vi "direct_tcpip.vi"() -> ()   [LabVIEW 2013]
uses:
  <vilib>/Utility/error.llb/DialogType.ctl
  libssh2/libssh2_init_default.vi
  libssh2/libssh2_session_handshake_tcp.vi
  libssh2/libssh2.lvlib
panel:
  in  "stop":bool
  out "error out":errorcluster
  in  "remote_destport":i32=2222
  in  "remote_desthost":string="localhost"
  in  "local_listenport":u16=4444
  in  "local_listenip":string="localhost"
  in  "server_ip":string="127.0.0.1"
  in  "password":string
  in  "username":string
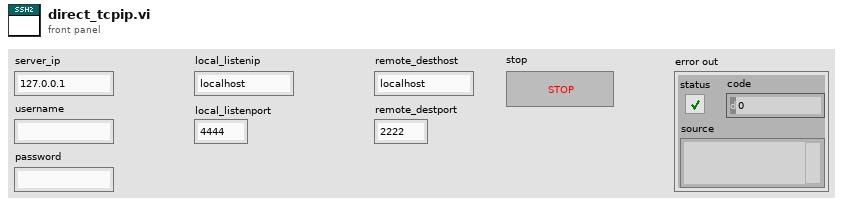
[diagram p1: front panel]
types:
  T1 = typedef "libssh2.lvlib/Session Refnum.ctl" = refnum<k1>
  T2 = typedef "libssh2.lvlib/Channel Refnum.ctl" = refnum<k1>
  T3 = enum16{"Standard", "Buffered", "CRLF", "Immediate"}
  T4 = typedef "DialogType.ctl" = u16
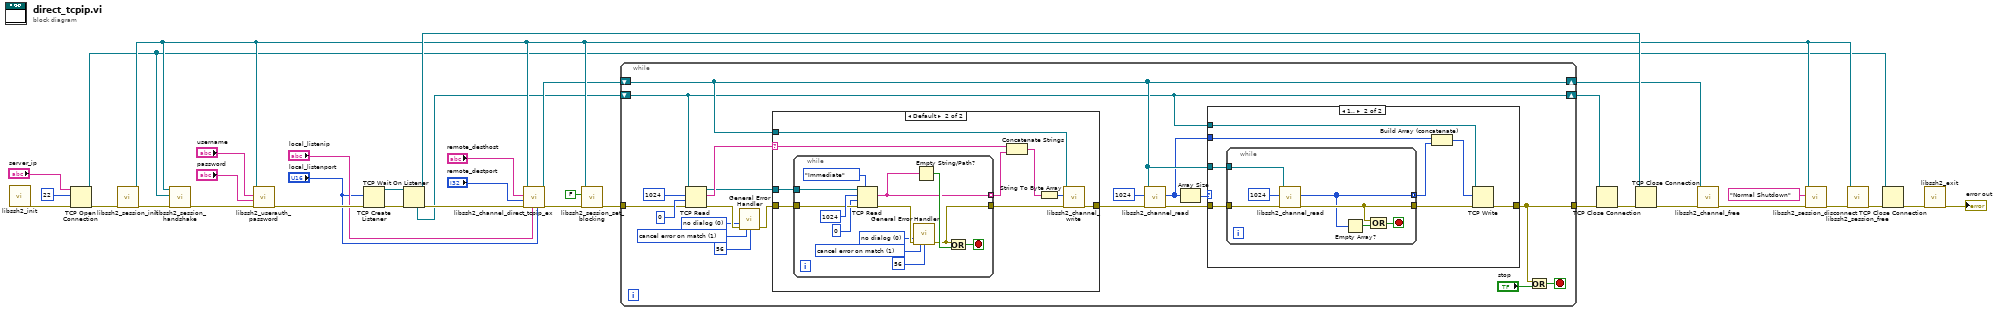
[diagram p0: block diagram]
diagram:
  n1 = call-poly "libssh2_init.vi"() -> ("error out"=w35:errorcluster)  [unwired: 11 in]
  n2 = TCP Open Connection(address="server_ip", remote port or service name=u16 22, error in (no error)=w35) -> (connection ID=w2:refnum<k5>, error out=w32:errorcluster)  [unwired: 2 in]
  n3 = call "libssh2_session_init.vi"("error in (no error)"=w32) -> ("error out"=w1:errorcluster, "session"=w18:T1)  [unwired: 9 in]
  n4 = call-poly "libssh2_session_handshake.vi"("error in (no error)"=w1, "tcp connection"=w2, "session"=w18) -> ("error out"=w31:errorcluster)  [unwired: 8 in]
  n5 = call "libssh2_userauth_password.vi"("error in (no error)"=w31, "password"="password", "username"="username", "session"=w18) -> ("error out"=w30:errorcluster)  [unwired: 7 in]
  n6 = TCP Create Listener(8:w30, 10:"local_listenport") -> (0:w17:errorcluster, 3:w12:refnum<k5>)  [unwired: 3 in, 1 out]
  n7 = TCP Wait On Listener(8:w17, 11:w12) -> (0:w27:errorcluster, 3:w19:refnum<k5>, 4:w5:refnum<k5>)  [unwired: 2 in, 2 out]
  n8 = call "libssh2_channel_direct_tcpip_ex.vi"("sport"="local_listenport", "shost"="local_listenip", "error in (no error)"=w27, "port"="remote_destport", "host"="remote_desthost", "session"=w18) -> ("error out"=w26:errorcluster, "channel"=w8:T2)  [unwired: 4 in]
  n9 = call "libssh2_session_set_blocking.vi"("error in (no error)"=w26, "blocking"=FALSE, "session"=w18) -> ("error out"=w10:errorcluster)  [unwired: 8 in]
  n10 = while {
    tunnel: w10 -> [w47]
    tunnel: [w43] -> w9
    shift-right: [w49] -> w6
    shift-left: w8 -> [w49]
    shift-right: [w44] -> w4
    shift-left: w5 -> [w44]
    stop <- w41 stop-if-true
    w38 = T4 0 items=["no dialog", "OK message", "continue or stop message", "OK message + warnings", "continue/stop + warnings"] ("type of dialog (OK msg:1)")
    w40 = 1 items=["no exception", "cancel error on match", "set error on match"] ("[exception action] (none:0)")
    n11 = TCP Read(connection ID=w44, bytes to read=1024, error in (no error)=w47, 9:0 ("timeout ms (25000)")) -> (connection ID out=w45:refnum<k5>, data out=w54:string, error out=w48:errorcluster)  [unwired: 1 in]
    n12 = call <vilib>:"General Error Handler.vi"("type of dialog (OK msg:1)"=w38, "error in (no error)"=w48, "[exception action] (none:0)"=w40, "[exception code]"=56 ("specific error code to clear (0: all)")) -> ("error out"=w46:errorcluster)  [unwired: 7 in, 4 out]
    n13 = case shown="Default" w54 {
      selector: w54 -> [_ w75]
      tunnel: [w72 w78] -> w51
      tunnel: w45 -> [_ w81]
      tunnel: w46 -> [w72 w80]
      tunnel: w49 -> [_ w77]
      frame "" {
      }
      frame Default {
        n14 = while {
          tunnel: [w86] -> w79
          tunnel: w81 -> [w92]
          tunnel: w80 -> [w89]
          tunnel: [w85] -> w76 mode=indexing
          stop <- w90 stop-if-true
          w83 = T4 0 items=["no dialog", "OK message", "continue or stop message", "OK message + warnings", "continue/stop + warnings"] ("type of dialog (OK msg:1)")
          w84 = 1 items=["no exception", "cancel error on match", "set error on match"] ("[exception action] (none:0)")
          n15 = TCP Read(connection ID=w92, bytes to read=1024, error in (no error)=w89, 7:T3."Immediate" ("mode (standard)"), 9:0 ("timeout ms (25000)")) -> (data out=w85:string, error out=w87:errorcluster)  [unwired: 1 out]
          n16 = call <vilib>:"General Error Handler.vi"("type of dialog (OK msg:1)"=w83, "error in (no error)"=w87, "[exception action] (none:0)"=w84, "[exception code]"=56 ("specific error code to clear (0: all)")) -> ("error out"=w86:errorcluster)  [unwired: 7 in, 4 out]
          n17 = Empty String/Path?(string/path=w85) -> (empty?=w91:bool)
          n18 = Or(x=w86, y=w91) -> (x .or. y?=w90:bool)
        }
        n19 = Concatenate Strings(w75, w76) -> (w74:string)
        n20 = String To Byte Array(string=w74) -> (unsigned byte array=w73:u8[])
        n21 = call "libssh2_channel_write.vi"("error in (no error)"=w79, "buffer"=w73, "channel"=w77) -> ("error out"=w78:errorcluster)  [unwired: 7 in, 1 out]
      }
    }
    n22 = call "libssh2_channel_read.vi"("error in (no error)"=w51, "buffer length"=1024 ("buflen"), "channel"=w49) -> ("error out"=w50:errorcluster, "buffer"=w36:u8[])  [unwired: 7 in]
    n23 = Array Size(array=w36) -> (size(s)=w37:i32)
    n24 = case shown="1.." w37 {
      tunnel: [w56 w62] -> w43
      tunnel: w49 -> [_ w64]
      tunnel: w44 -> [_ w61]
      tunnel: w50 -> [w56 w63]
      tunnel: w36 -> [_ w60]
      frame Default {
      }
      frame 1.. {
        n25 = while {
          tunnel: w64 -> [w67]
          tunnel: w63 -> [w68]
          tunnel: [w65] -> w59 mode=concatenating
          tunnel: [w66] -> w57
          stop <- w71 stop-if-true
          n26 = call "libssh2_channel_read.vi"("error in (no error)"=w68, "buffer length"=1024 ("buflen"), "channel"=w67) -> ("error out"=w66:errorcluster, "buffer"=w65:u8[])  [unwired: 7 in]
          n27 = Empty Array?(array=w65) -> (empty?=w70:bool)
          n28 = Compound Arithmetic op=OR(w66, w70) -> (w71:bool)
        }
        n29 = Build Array (concatenate)(w60, w59) -> (w58:u8[])
        n30 = TCP Write(connection ID=w61, data in=w58, error in (no error)=w57) -> (error out=w62:errorcluster)  [unwired: 1 in, 2 out]
      }
    }
    n31 = Or(x=w43, y="stop") -> (x .or. y?=w41:bool)
  }
  n32 = TCP Close Connection(connection ID=w4, error in (no error)=w9) -> (error out=w11:errorcluster)  [unwired: 1 in, 1 out]
  n33 = TCP Close Connection(connection ID=w19, error in (no error)=w11) -> (error out=w22:errorcluster)  [unwired: 1 in, 1 out]
  n34 = call "libssh2_channel_free.vi"("error in (no error)"=w22, "channel"=w6) -> ("error out"=w25:errorcluster)  [unwired: 9 in]
  n35 = call "libssh2_session_disconnect.vi"("error in (no error)"=w25, "description"="Normal Shutdown", "session"=w18) -> ("error out"=w23:errorcluster)  [unwired: 8 in]
  n36 = call "libssh2_session_free.vi"("error in (no error)"=w23, "session"=w18) -> ("error out"=w21:errorcluster)  [unwired: 9 in]
  n37 = TCP Close Connection(connection ID=w2, error in (no error)=w21) -> (error out=w7:errorcluster)  [unwired: 1 in, 1 out]
  n38 = call "libssh2_exit.vi"("error in (no error)"=w7) -> ("error out"=→"error out":errorcluster)  [unwired: 10 in]
